vi "ma_SML Magnitude and Phase.vi"(2 "settings":T1, 3 "FFT spectrum":cluster{"f0":dbl, "df":dbl, "spectrum":cdb[]} {"spectrum" format="%.2f"; "df" format="%.2f"; "f0" format="%.2f"}) -> (0 "phase":cluster{"f0":dbl, "df":dbl, "Y":dbl[]} {"Y" format="%.2f"; "df" format="%.2f"; "f0" format="%.2f"}, 1 "magnitude":cluster{"f0":dbl, "df":dbl, "Y":dbl[]} {"Y" format="%.2f"; "df" format="%.2f"; "f0" format="%.2f"})   [LabVIEW 2020, in "NI_MAPro.lvlib"]
uses:
  NI_MAPro.lvlib
  NI_AALPro.lvlib
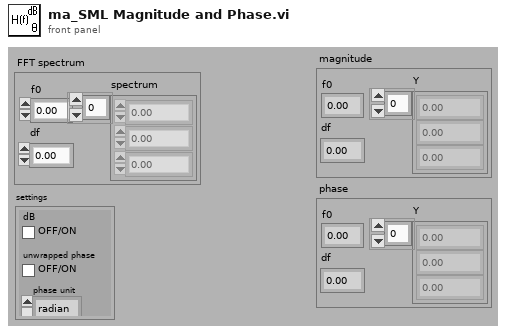
[diagram p1: front panel]
types:
  T1 = cluster{"dB":bool, "unwrapped phase":bool, "phase unit":enum16{"radian", "degree"}}
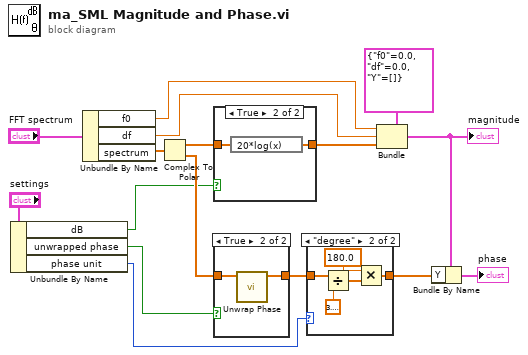
[diagram p0: block diagram]
diagram:
  n1 = Unbundle By Name("settings") -> ("dB"=w3:bool, "unwrapped phase"=w2:bool, "phase unit"=w1:enum16{"radian", "degree"})
  n2 = Unbundle By Name("FFT spectrum") -> ("f0"=w13:dbl, "df"=w12:dbl, "spectrum"=w15:cdb[])
  n3 = Complex To Polar(r * e^(i*theta)=w15) -> (r=w14:dbl[], theta=w10:dbl[])
  n4 = case shown="True" w3 {
    tunnel: w14 -> [w17 w19]
    tunnel: [w17 w18] -> w11
    frame False {
    }
    frame True {
      n5 = expression code="20*log(x)"(w19) -> (w18:dbl[])
    }
  }
  n6 = case shown="True" w2 {
    tunnel: w10 -> [w20 w22]
    tunnel: [w20 w21] -> w9
    frame False {
    }
    frame True {
      n7 = call "Unwrap Phase.vi"("Phase"=w22) -> ("Unwrapped Phase"=w21:dbl[])  [unwired: 1 in, 9 out]
    }
  }
  n8 = case shown="\"degree\"" w1 {
    tunnel: [w23 w25] -> w6
    tunnel: w9 -> [w23 w28]
    frame "radian", Default {
    }
    frame "degree" {
      n9 = Divide(x=w28, y=3.141592653589793) -> (x/y=w26:dbl[])
      n10 = Multiply(x=180.0, y=w26) -> (x*y=w25:dbl[])
    }
  }
  n11 = Bundle(cluster=cluster{"f0":dbl, "df":dbl, "Y":dbl[]} {"f0"=0.0, "df"=0.0, "Y"=[]} ("magnitude"), "f0"=w13, "df"=w12, "Y"=w11) -> (w8:cluster{"f0":dbl, "df":dbl, "Y":dbl[]})
  "magnitude" <- w8
  n12 = Bundle By Name(cluster=w8, "Y"=w6) -> (→"phase":cluster{"f0":dbl, "df":dbl, "Y":dbl[]})
